vi "Write Roles.vi"(8 "error in (no error)":errorcluster, 10 "Roles":T1, 11 "BallChallengePlayVSS in":refnum<class "BallChallengePlayVSS.lvclass">) -> (0 "error out":errorcluster, 3 "BallChallengePlayVSS out":refnum<class "BallChallengePlayVSS.lvclass">)   [LabVIEW 2020, in "BallChallengePlayVSS.lvclass"]
uses:
  BallChallengePlayVSS.lvclass
  HaltRole_class/HaltRole.lvclass
  BallChallengerAttackerRoleVSS_class/BallChallengerAttackerRoleVSS.lvclass
  BallChallengePlayVSS.lvclass/BallChallengePlayVSS.ctl
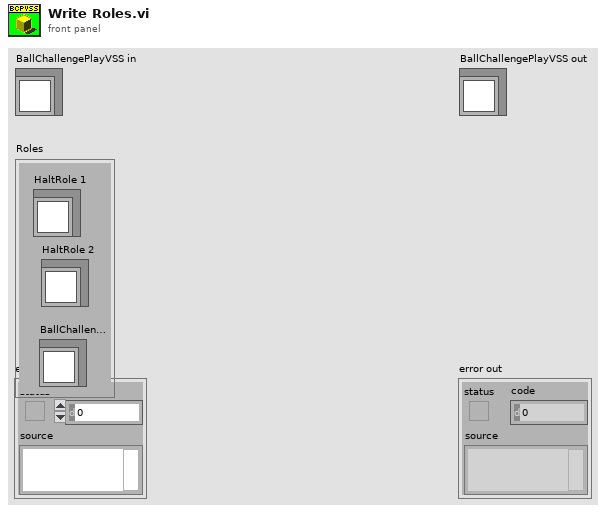
[diagram p1: front panel]
types:
  T1 = cluster{"HaltRole 1":refnum<class "HaltRole.lvclass">, "HaltRole 2":refnum<class "HaltRole.lvclass">, "BallChallengerAttackerRoleVSS":refnum<class "BallChallengerAttackerRoleVSS.lvclass">}
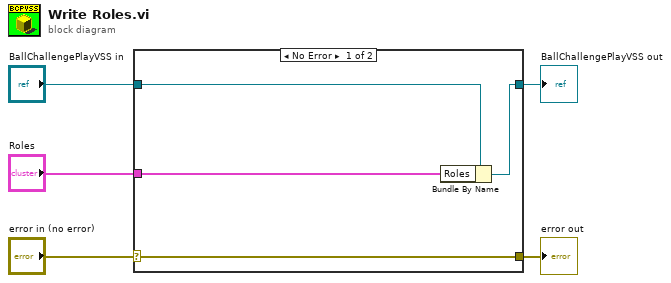
[diagram p0: block diagram]
diagram:
  n1 = case shown="No Error" "error in (no error)" {
    selector: "error in (no error)" -> [w9 w10]
    tunnel: [w9 w10] -> w4
    tunnel: [w7 w11] -> w2
    tunnel: "BallChallengePlayVSS in" -> [w8 w11]
    tunnel: "Roles" -> [w6 _]
    frame No Error {
      n2 = Bundle By Name(cluster=w8, "Roles"=w6) -> (w7:refnum<class "BallChallengePlayVSS.lvclass">)
    }
    frame Error {
    }
  }
  "error out" <- w4
  "BallChallengePlayVSS out" <- w2
